vi "河内塔-全局.vi"() -> ()   [LabVIEW 2016]
panel:
  out "数组":cluster{"n":u8, "From":string, "To":string}[](array[cluster])
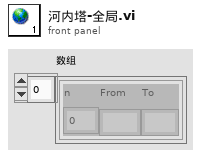
[diagram p1: front panel]
diagram:
